vi "Get State.vi"(2 "Data":T3) -> (5 "Redraw Scene":bool, 6 "Scene":refnum<vi>, 8 "Global Events":T1, 9 "Display":u8, 10 "State":T2)   [LabVIEW 2020, in "AR Example.lvlib"]
uses:
  AR Example.lvlib
  Data.ctl
  g_ar_toolkit.capture/CameraManager/CameraManager.lvclass
  Tab Control.ctl
  State.ctl
  Global Events.ctl
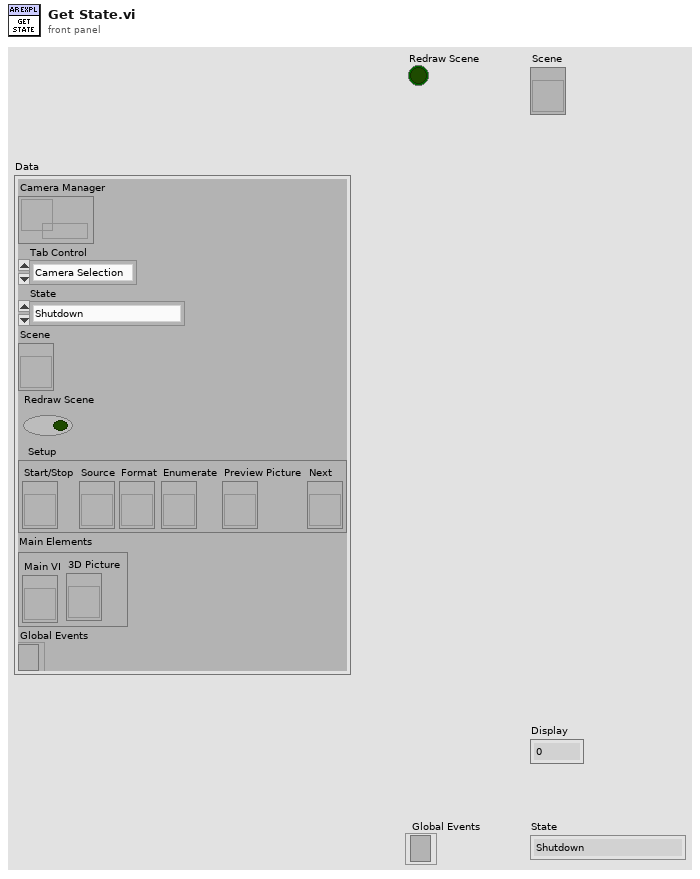
[diagram p1: front panel]
types:
  T1 = typedef "AR Example.lvlib/Global Events.ctl" = refnum<event-registration>
  T2 = typedef "AR Example.lvlib/State.ctl" = enum16{"Shutdown", "Initialize", "Select Camera"}
  T3 = typedef "AR Example.lvlib/Data.ctl" = cluster{"Camera Manager":refnum<data-value>, "Tab Control":T4, "State":T2, "Scene":refnum<vi>, "Redraw Scene":bool, "Setup":cluster{"Start/Stop":refnum<vi>, "Source":refnum<vi>, "Format":refnum<vi>, "Enumerate":refnum<vi>, "Preview Picture":refnum<vi>, "Next":refnum<vi>}, "Main Elements":cluster{"Main VI":refnum<vi>, "3D Picture":refnum<vi>}, "Global Events":T1}
  T4 = typedef "AR Example.lvlib/Tab Control.ctl" = enum8{"Camera Selection"}
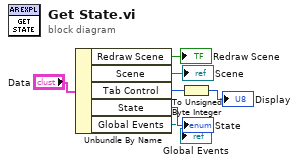
[diagram p0: block diagram]
diagram:
  n1 = Unbundle By Name("Data") -> ("Redraw Scene"=→"Redraw Scene":bool, "Scene"=→"Scene":refnum<vi>, "Tab Control"=w4:T4, "State"=→"State":T2, "Global Events"=→"Global Events":T1)
  n2 = To Unsigned Byte Integer(number=w4) -> (unsigned 8bit integer=→"Display":u8)
